vi "json Insert json Array - string path.vi"(8 "error in (no error)":errorcluster, 9 "anything":refnum<class "JSON Document.lvclass">[](array[class]), 10 "path":string, 11 "JSON Document in":refnum<class "JSON Document.lvclass">) -> (0 "error out":errorcluster, 1 "replaced?":bool, 3 "JSON Document out":refnum<class "JSON Document.lvclass">)   [LabVIEW 2015, in "JSON Document.lvclass"]
uses:
  JSON Document.lvclass
  json Insert json - string path.vi
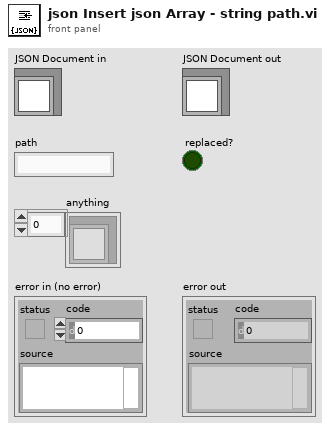
[diagram p1: front panel]
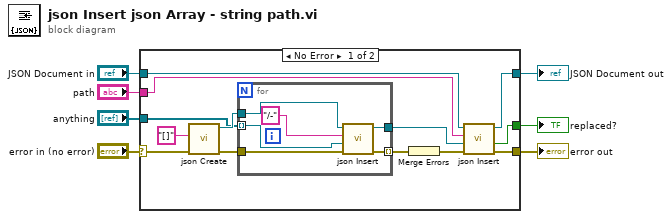
[diagram p0: block diagram]
diagram:
  n1 = case shown="No Error" "error in (no error)" {
    selector: "error in (no error)" -> [w8 w28]
    tunnel: [w20 w28] -> w6
    tunnel: [w13 w27] -> w4
    tunnel: "JSON Document in" -> [w10 w27]
    tunnel: "anything" -> [w16 _]
    tunnel: "path" -> [w9 _]
    tunnel: [w19 _] -> w1
    frame No Error {
      n2 = call "json Create.vi"("error in (no error)"=w8, "JSON String"="[]") -> ("error out"=w12:errorcluster, "JSON Document out"=w17:refnum<class "JSON Document.lvclass">)  [unwired: 8 in]
      n3 = for {
        tunnel: w17 -> [w26]
        tunnel: w16 -> [w25] mode=indexing
        tunnel: w12 -> [w24]
        tunnel: [w23] -> w15 mode=indexing
        tunnel: [w22] -> w11
        n4 = call-poly "json Insert.vi"("error in (no error)"=w24, "anything"=w25, "path"="/-" ("initial string"), "JSON Document in"=w26) -> ("error out"=w23:errorcluster, "JSON Document out"=w22:refnum<class "JSON Document.lvclass">)  [unwired: 5 in, 1 out]
      }
      n5 = Merge Errors(w15) -> (w14:errorcluster)
      n6 = call-poly "json Insert.vi"("error in (no error)"=w14, "anything"=w11, "path"=w9, "JSON Document in"=w10) -> ("error out"=w20:errorcluster, "replaced?"=w19:bool, "JSON Document out"=w13:refnum<class "JSON Document.lvclass">)  [unwired: 5 in]
    }
    frame Error {
    }
  }
  "error out" <- w6
  "JSON Document out" <- w4
  "replaced?" <- w1
